vi "CMD_Loop.vi"() -> ()   [LabVIEW 2020, in "Template_CMD.lvlib"]
uses:
  Template_CMD.lvlib
  Cluster_CMD_CMD_Data.ctl
  ENUM_CMD_State.ctl
  ENUM_CMD_Action.ctl
  RoboRIO Utilities/Global_STOP.vi
  Global_CMD_CMD_Data In.vi
  Global_CMD_Data Out.vi
panel:
  out "Input Data":T1
  out "Output DBL Data":dbl
  out "Cycle Time (S)":dbl format="%.3g"
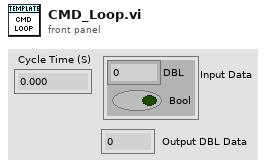
[diagram p1: front panel]
types:
  T1 = typedef "Template_CMD.lvlib/Cluster_CMD_CMD_Data.ctl" = cluster{"DBL":dbl, "Bool":bool}
  T2 = typedef "Template_CMD.lvlib/ENUM_CMD_State.ctl" = enum16{"Startup", "Idle", "Shutdown"}
  T3 = typedef "Template_CMD.lvlib/ENUM_CMD_Action.ctl" = enum16{"No Action", "Reset Time", "Reset All", "Action A", "Action B"}
  T4 = cluster{"State":T2, "Previous State":T2, "Current Time":timestamp, "Previous Time":timestamp, "Start Time":timestamp, "Target Time (ms)":u32, "Cycle Time(S)":dbl, "CMD Input":T1, "Output DBL":dbl}
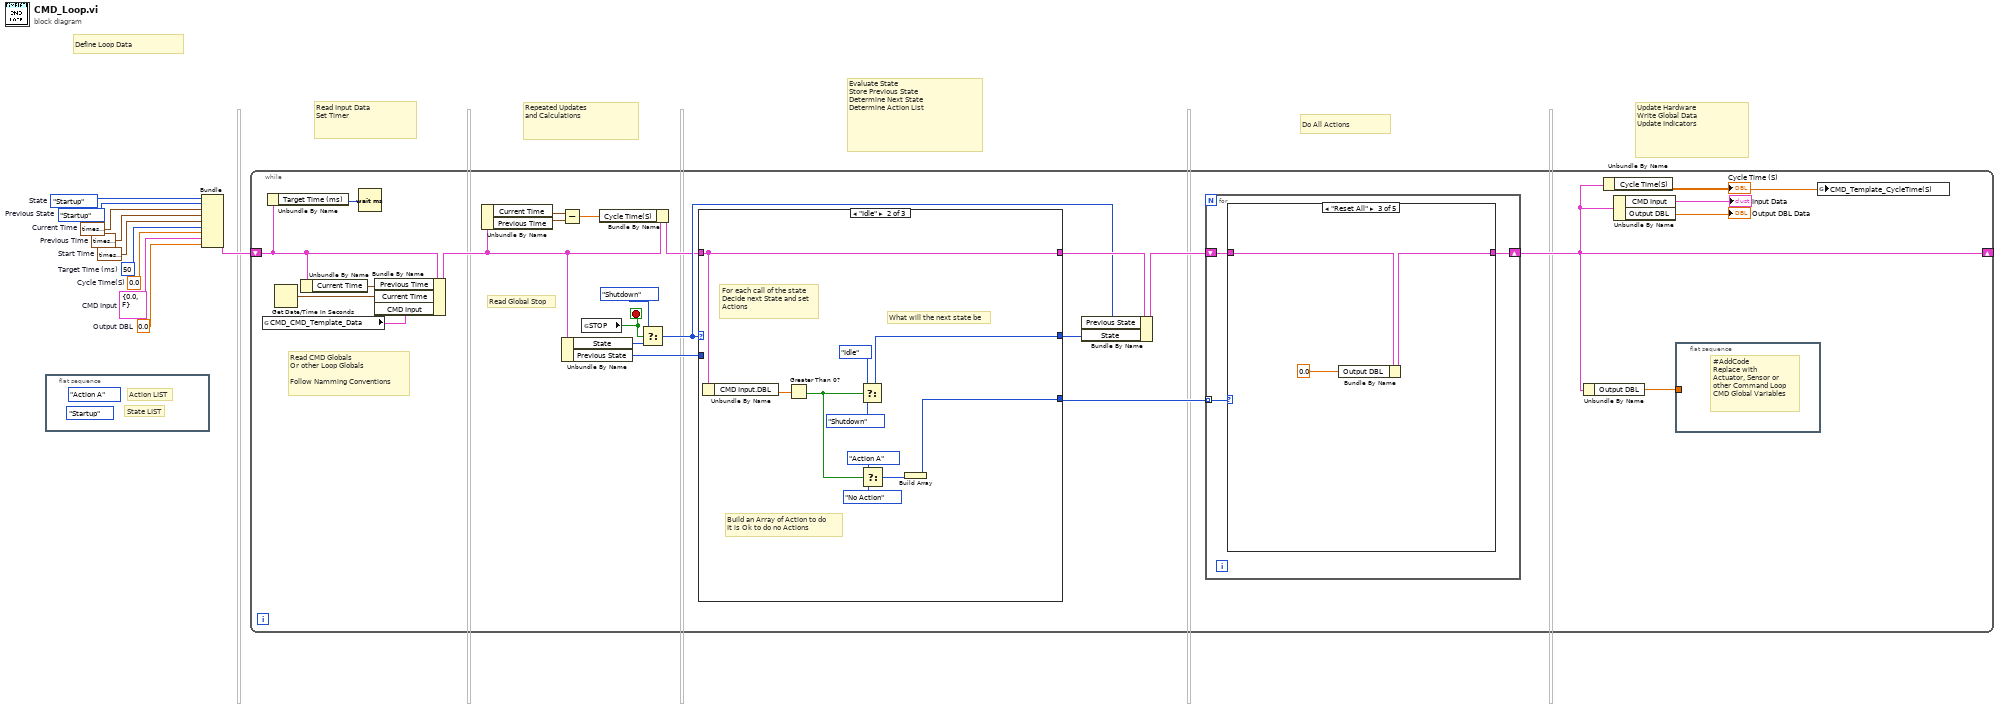
[diagram p0: block diagram]
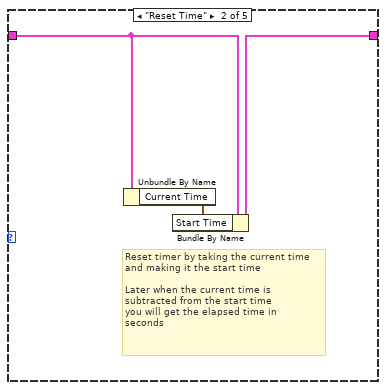
[diagram p3: hidden frame]
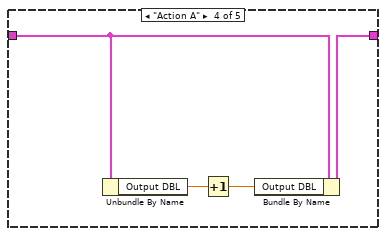
[diagram p4: hidden frame]
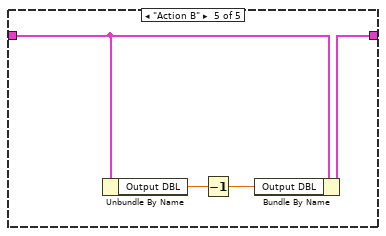
[diagram p5: hidden frame]
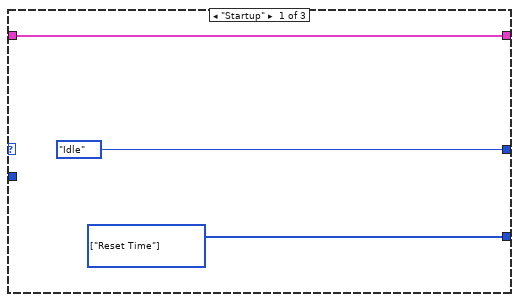
[diagram p6: hidden frame]
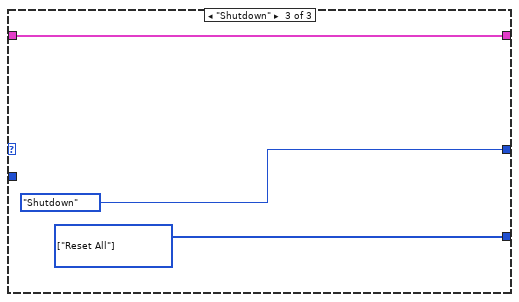
[diagram p7: hidden frame]
diagram:
  w1 = 0.0  # Cycle Time(S)
  w2 = ENUM_CMD_State."Startup"  # Previous State
  w3 = timestamp(0 s since 1904-01-01)  # Previous Time
  w4 = u32 50  # Target Time (ms)
  w5 = 0.0  # Output DBL
  w6 = T1 {"DBL"=0.0, "Bool"=FALSE}  # CMD Input
  w7 = timestamp(0 s since 1904-01-01)  # Start Time
  w8 = timestamp(0 s since 1904-01-01)  # Current Time
  w9 = ENUM_CMD_State."Startup"  # State
  # "Define Loop Data"
  # "Repeated Updates\nand Calculations"
  # "Read Input Data\nSet Timer"
  # "Evaluate State\nStore Previous State\nDetermine Next State\nDetermine Action List"
  # "Do All Actions"
  # "Update Hardware\nWrite Global Data\nUpdate Indicators"
  n1 = flat-sequence {
    frame #0 {
      (unwired) ENUM_CMD_State."Startup" ("State")
      (unwired) ENUM_CMD_Action."Action A" ("Action")
      # "State LIST"
      # "Action LIST"
    }
  }
  n2 = Bundle("State"=w9, "Previous State"=w2, "Current Time"=w8, "Previous Time"=w3, "Start Time"=w7, "Target Time (ms)"=w4, "Cycle Time(S)"=w1, "CMD Input"=w6, "Output DBL"=w5) -> (w10:T4)  [unwired: 1 in]
  n3 = while {
    shift-right: [w13] -> _
    shift-left: w10 -> [w25]
    stop <- w30 stop-if-true
    # "Read CMD Globals\nOr other Loop Globals\n\nFollow Namming Conventions"
    # "Read Global Stop"
    n4 = global read "Global_CMD_CMD_Data In.vi" "CMD_CMD_Template_Data"() -> (w14:T1)
    n5 = Unbundle By Name(w25) -> ("Target Time (ms)"=w27:u32)
    n6 = Get Date/Time In Seconds() -> (seconds since 1Jan1904=w34:timestamp)
    n7 = Unbundle By Name(w25) -> ("Current Time"=w26:timestamp)
    n8 = Wait (ms)(milliseconds to wait=w27) -> ()  [unwired: 1 out]
    n9 = Bundle By Name(cluster=w25, "Previous Time"=w26, "Current Time"=w34, "CMD Input"=w14) -> (w19:T4)
    n10 = Unbundle By Name(w19) -> ("Current Time"=w20:timestamp, "Previous Time"=w21:timestamp)
    n11 = Subtract(x=w20, y=w21) -> (x-y=w17:dbl)
    n12 = Unbundle By Name(w19) -> ("State"=w28:T2, "Previous State"=w24:T2)
    n13 = global read "Global_STOP.vi" "STOP"() -> (w30:bool)
    n14 = Bundle By Name(cluster=w19, "Cycle Time(S)"=w17) -> (w18:T4)
    n15 = Select(t=ENUM_CMD_State."Shutdown" ("State"), s=w30, f=w28) -> (s? t:f=w22:T2)
    n16 = case shown="\"Idle\"" w22 {
      tunnel: w18 -> [w55 w65 w68]
      tunnel: [w55 w65 w68] -> w32
      tunnel: [ENUM_CMD_State."Idle" ("State") w63 ENUM_CMD_State."Shutdown" ("State")] -> w31
      tunnel: [w54 w56 w66] -> w16
      tunnel: w24 -> [_ _ _]
      frame "Startup" {
        w54 = T3[] [enum."Reset Time"] items=["No Action", "Reset Time", "Reset All", "Action A", "Action B"] ("Actions")
      }
      frame "Idle" {
        # "For each call of the state\nDecide next State and set\nActions"
        # "What will the next state be"
        # "Build an Array of Action to do\nIt is Ok to do no Actions"
        n17 = Unbundle By Name(w65) -> ("CMD Input.DBL"=w64:dbl)
        n18 = Greater Than 0?(x=w64) -> (x > 0?=w58:bool)
        n19 = Select(t=ENUM_CMD_State."Idle" ("State"), s=w58, f=ENUM_CMD_State."Shutdown" ("State")) -> (s? t:f=w63:T2)
        n20 = Select(t=ENUM_CMD_Action."Action A" ("Action"), s=w58, f=ENUM_CMD_Action."No Action" ("Action")) -> (s? t:f=w57:T3)
        n21 = Build Array(w57) -> (w56:T3[])
      }
      frame "Shutdown" {
        w66 = T3[] [enum."Reset All"] items=["No Action", "Reset Time", "Reset All", "Action A", "Action B"] ("Actions")
      }
    }
    n22 = Bundle By Name(cluster=w32, "Previous State"=w22, "State"=w31) -> (w33:T4)
    n23 = for {
      tunnel: w16 -> [w37] mode=indexing
      shift-right: [w36] -> w13
      shift-left: w33 -> [w35]
      n24 = case shown="\"Reset All\"" w37 {
        tunnel: w35 -> [w38 w41 w44 w47 w51]
        tunnel: [w38 w40 w43 w46 w50] -> w36
        frame "No Action" {
        }
        frame "Reset Time" {
          # "Reset timer by taking the current time\nand making it the start time\n\nLater when the current time is \nsubtracted from the start time\nyou will get the elapsed time in \nseconds"
          n25 = Unbundle By Name(w41) -> ("Current Time"=w39:timestamp)
          n26 = Bundle By Name(cluster=w41, "Start Time"=w39) -> (w40:T4)
        }
        frame "Reset All" {
          n27 = Bundle By Name(cluster=w44, "Output DBL"=0.0 ("FG Write Value")) -> (w43:T4)
        }
        frame "Action A" {
          n28 = Unbundle By Name(w47) -> ("Output DBL"=w48:dbl)
          n29 = Increment(x=w48) -> (x+1=w45:dbl)
          n30 = Bundle By Name(cluster=w47, "Output DBL"=w45) -> (w46:T4)
        }
        frame "Action B" {
          n31 = Unbundle By Name(w51) -> ("Output DBL"=w52:dbl)
          n32 = Decrement(x=w52) -> (x-1=w49:dbl)
          n33 = Bundle By Name(cluster=w51, "Output DBL"=w49) -> (w50:T4)
        }
      }
    }
    n34 = Unbundle By Name(w13) -> ("Output DBL"=w12:dbl)
    n35 = Unbundle By Name(w13) -> ("Cycle Time(S)"=w11:dbl)
    "Cycle Time (S)" <- w11
    n36 = Unbundle By Name(w13) -> ("CMD Input"=→"Input Data":T1, "Output DBL"=→"Output DBL Data":dbl)
    n37 = flat-sequence {
      tunnel: w12 -> [_]
      frame #0 {
        # "#AddCode\nReplace with\nActuator, Sensor or\nother Command Loop\nCMD Global Variables"
      }
    }
    n38 = global write "Global_CMD_Data Out.vi" "CMD_Template_CycleTime(S)"(w11) -> ()
  }
